vi "Get Measurement Descriptions.vi"(8 "error in (no error)":errorcluster, 11 "Measurement Data in":refnum<class "Measurement Data.lvclass">) -> (0 "error out":errorcluster, 2 "Measurement Step Descriptions":T1[](array[typedef]), 3 "Measurement Data out":refnum<class "Measurement Data.lvclass">)   [LabVIEW 2018, in "Measurement Data.lvlib" / "Measurement Data.lvclass"]
uses:
  Measurement Data.lvclass
  Controls/Measurement Description.ctl
  Plugins/String Database.lvlibp/String Database.lvclass
  Controls/Measurement Position.ctl
  Measurement Data.lvclass/Measurement Data.ctl
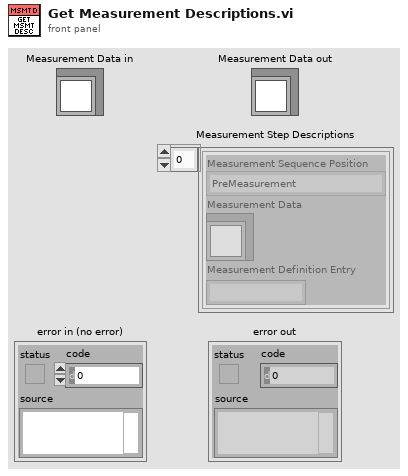
[diagram p1: front panel]
types:
  T1 = typedef "Measurement Data.lvlib/Measurement Data.lvclass/Measurement Description.ctl" = cluster{"Measurement Sequence Position":T2, "Measurement Data":refnum<class "String Database.lvclass">, "Measurement Definition Entry":string}
  T2 = typedef "Measurement Data.lvlib/Measurement Data.lvclass/Measurement Position.ctl" = enum16{"PreMeasurement", "MainMeasurement", "PostMeasurement"}
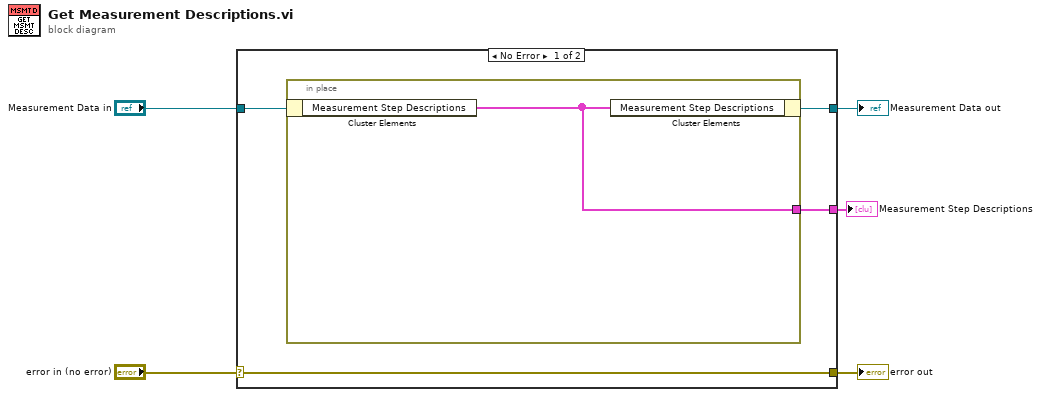
[diagram p0: block diagram]
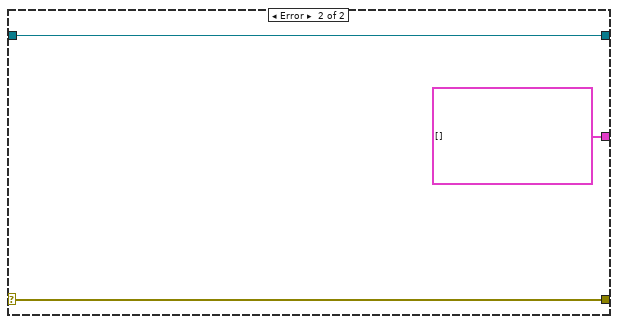
[diagram p2: hidden frame]
diagram:
  n1 = case shown="No Error" "error in (no error)" {
    selector: "error in (no error)" -> [w9 w13]
    tunnel: [w9 w13] -> w4
    tunnel: [w6 w12] -> w2
    tunnel: "Measurement Data in" -> [w8 w12]
    tunnel: [w7 T1[] [] ("Measurement Step Descriptions")] -> w1
    frame No Error {
      n2 = in-place {
        in-place-border: [w10] -> w7
        n3 = in-place-cluster #1(w8) -> ("Measurement Step Descriptions"=w10:T1[])
        n4 = in-place-cluster #1("Measurement Step Descriptions"=w10) -> (w6:refnum<class "Measurement Data.lvclass">)
      }
    }
    frame Error {
    }
  }
  "error out" <- w4
  "Measurement Data out" <- w2
  "Measurement Step Descriptions" <- w1
